vi "SimulationSubVI.vi"(0 "varIn":T1={"nodes"=[], "edges"=[], "nodeSelected"=-1, "bPressed"=FALSE, "NodeRef"=[]} {"edges"."len" format="%.2f"; "nodes"."h" format="%.2f"; "nodes"."w" format="%.2f"; "nodes"."dy" format="%.2f"; "nodes"."dx" format="%.2f"; "nodes"."y" format="%.2f"; "nodes"."x" format="%.2f"}) -> (14 "varOut":T1={"nodes"=[], "edges"=[], "nodeSelected"=-1, "bPressed"=FALSE, "NodeRef"=[]} {"edges"."len" format="%.2f"; "nodes"."h" format="%.2f"; "nodes"."w" format="%.2f"; "nodes"."dy" format="%.2f"; "nodes"."dx" format="%.2f"; "nodes"."y" format="%.2f"; "nodes"."x" format="%.2f"})   [LabVIEW 2010]
uses:
  localVar.ctl
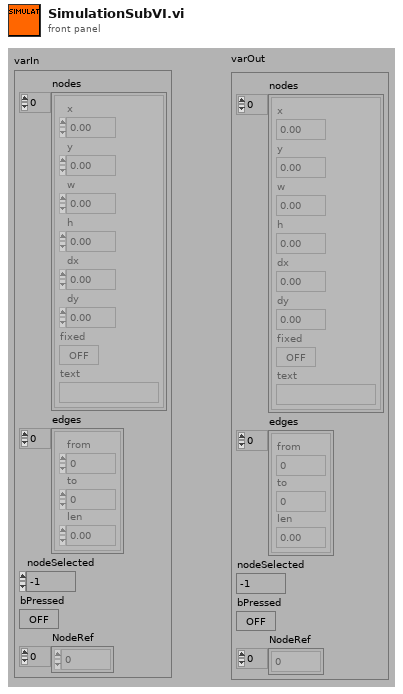
[diagram p1: front panel]
types:
  T1 = typedef "localVar.ctl" = cluster{"nodes":cluster{"x":dbl, "y":dbl, "w":dbl, "h":dbl, "dx":dbl, "dy":dbl, "fixed":bool, "text":string}[], "edges":cluster{"from":i32, "to":i32, "len":dbl}[], "nodeSelected":i32, "bPressed":bool, "NodeRef":u32[]}
  T2 = cluster{"x":dbl, "y":dbl, "w":dbl, "h":dbl, "dx":dbl, "dy":dbl, "fixed":bool, "text":string}[]
  T3 = cluster{"x":dbl, "y":dbl, "w":dbl, "h":dbl, "dx":dbl, "dy":dbl, "fixed":bool, "text":string}
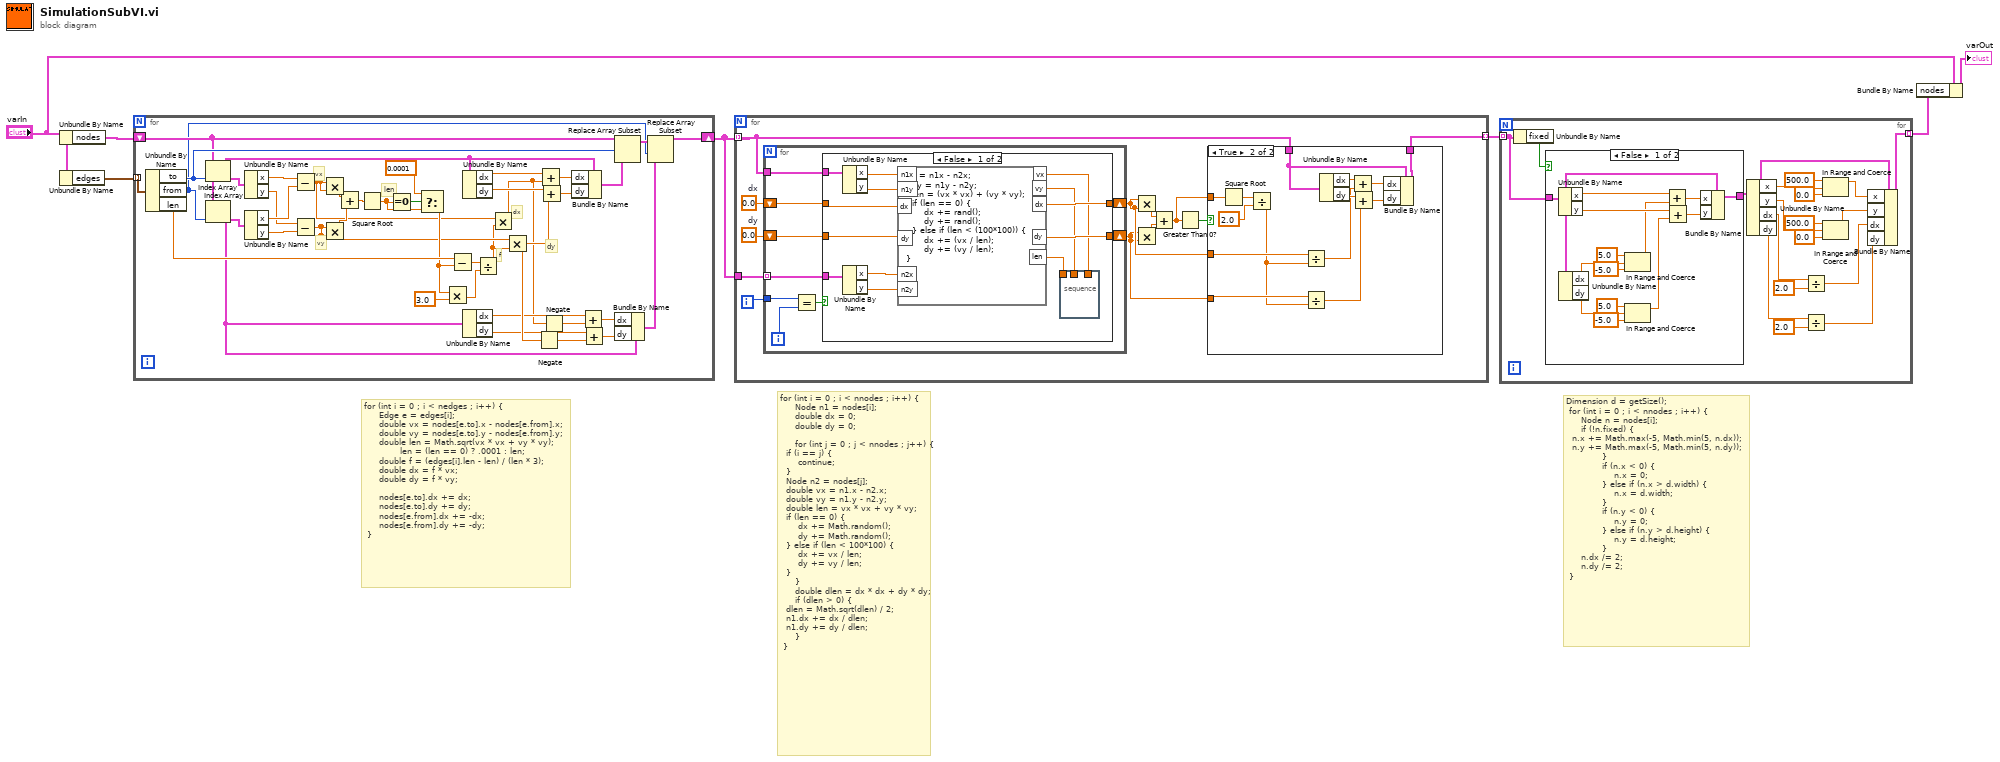
[diagram p0: block diagram]
diagram:
  # "Dimension d = getSize();\n\tfor (int i = 0 ; i < nnodes ; i++) {\n\t    Node n = nodes[i];\n\t    if (!n.fixed) {\n\t\tn.x += Math.max(-5, Math.min(5, n.dx));\n\t\tn.y += Math.max(-5, Math.min(5, n.dy));\n            }\n            if (n.x < 0) {\n                n.x = 0;\n            } else if (n.x > d.width) {\n                n.x = d.width;\n            }\n            if (n.y < 0) {\n                n.y = 0;\n            } else if (n.y > d.height) {\n                n.y = d.height;\n            }\n\t    n.dx /= 2;\n\t    n.dy /= 2;\n\t}"
  # "for (int i = 0 ; i < nnodes ; i++) {\n\t    Node n1 = nodes[i];\n\t    double dx = 0;\n\t    double dy = 0;\n\n\t    for (int j = 0 ; j < nnodes ; j++) {\n\t\tif (i == j) {\n\t\t    continue;\n\t\t}\n\t\tNode n2 = nodes[j];\n\t\tdouble vx = n1.x - n2.x;\n\t\tdouble vy = n1.y - n2.y;\n\t\tdouble len = vx * vx + vy * vy;\n\t\tif (len == 0) {\n\t\t    dx += Math.random();\n\t\t    dy += Math.random();\n\t\t} else if (len < 100*100) {\n\t\t    dx += vx / len;\n\t\t    dy += vy / len;\n\t\t}\n\t    }\n\t    double dlen = dx * dx + dy * dy;\n\t    if (dlen > 0) {\n\t\tdlen = Math.sqrt(dlen) / 2;\n\t\tn1.dx += dx / dlen;\n\t\tn1.dy += dy / dlen;\n\t    }\n\t}"
  # "for (int i = 0 ; i < nedges ; i++) {\n\t    Edge e = edges[i];\n\t    double vx = nodes[e.to].x - nodes[e.from].x;\n\t    double vy = nodes[e.to].y - nodes[e.from].y;\n\t    double len = Math.sqrt(vx * vx + vy * vy);\n            len = (len == 0) ? .0001 : len;\n\t    double f = (edges[i].len - len) / (len * 3);\n\t    double dx = f * vx;\n\t    double dy = f * vy;\n\n\t    nodes[e.to].dx += dx;\n\t    nodes[e.to].dy += dy;\n\t    nodes[e.from].dx += -dx;\n\t    nodes[e.from].dy += -dy;\n\t}"
  n1 = Unbundle By Name("varIn") -> ("nodes"=w6:T2)
  n2 = Unbundle By Name("varIn") -> ("edges"=w7:cluster{"from":i32, "to":i32, "len":dbl}[])
  n3 = for {
    tunnel: w7 -> [w47] mode=indexing
    shift-right: [w12] -> w1
    shift-left: w6 -> [w15]
    # "dy"
    # "dx"
    # "f"
    # "len"
    # "vy"
    # "vx"
    n4 = Unbundle By Name(w47) -> ("to"=w16:i32, "from"=w11:i32, "len"=w36:dbl)
    n5 = Index Array(array=w15, index=w16) -> (element=w31:T3)
    n6 = Index Array(array=w15, index=w11) -> (element=w17:T3)
    n7 = Unbundle By Name(w31) -> ("x"=w46:dbl, "y"=w43:dbl)
    n8 = Unbundle By Name(w17) -> ("x"=w45:dbl, "y"=w44:dbl)
    n9 = Subtract(x=w46, y=w45) -> (x-y=w26:dbl)
    n10 = Subtract(x=w43, y=w44) -> (x-y=w25:dbl)
    n11 = Multiply(x=w26, y=w26) -> (x*y=w41:dbl)
    n12 = Multiply(x=w25, y=w25) -> (x*y=w42:dbl)
    n13 = Add(x=w41, y=w42) -> (x+y=w40:dbl)
    n14 = Square Root(x=w40) -> (sqrt(x)=w37:dbl)
    n15 = Equal To 0?(x=w37) -> (x = 0?=w39:bool)
    n16 = Select(t=0.0001, s=w39, f=w37) -> (s? t:f=w34:dbl)
    n17 = Multiply(x=w34, y=3.0) -> (x*y=w32:dbl)
    n18 = Subtract(x=w36, y=w34) -> (x-y=w35:dbl)
    n19 = Unbundle By Name(w31) -> ("dx"=w30:dbl, "dy"=w29:dbl)
    n20 = Unbundle By Name(w17) -> ("dx"=w20:dbl, "dy"=w19:dbl)
    n21 = Divide(x=w35, y=w32) -> (x/y=w24:dbl)
    n22 = Multiply(x=w26, y=w24) -> (x*y=w18:dbl)
    n23 = Multiply(x=w25, y=w24) -> (x*y=w23:dbl)
    n24 = Negate(x=w23) -> (-x=w8:dbl)
    n25 = Add(x=w30, y=w18) -> (x+y=w28:dbl)
    n26 = Add(x=w29, y=w23) -> (x+y=w27:dbl)
    n27 = Negate(x=w18) -> (-x=w9:dbl)
    n28 = Bundle By Name(cluster=w31, "dx"=w28, "dy"=w27) -> (w14:T3)
    n29 = Add(x=w20, y=w9) -> (x+y=w21:dbl)
    n30 = Add(x=w19, y=w8) -> (x+y=w22:dbl)
    n31 = Replace Array Subset(array=w15, new element=w14, index=w16) -> (w13:T2)
    n32 = Bundle By Name(cluster=w17, "dx"=w21, "dy"=w22) -> (w10:T3)
    n33 = Replace Array Subset(array=w13, new element=w10, index=w11) -> (w12:T2)
  }
  n34 = for {
    tunnel: w1 -> [w48] mode=indexing
    tunnel: [w52] -> w3 mode=indexing
    tunnel: w1 -> [w49]
    i -> [w59]
    w58 = 0.0  # dx
    w57 = 0.0  # dy
    n35 = for {
      tunnel: w59 -> [w83]
      shift-right: [w80] -> w51
      shift-left: w58 -> [w79]
      shift-right: [w78] -> w50
      shift-left: w57 -> [w77]
      tunnel: w49 -> [w76] mode=indexing
      tunnel: w48 -> [w75]
      i -> [w82]
      n36 = Equal?(x=w83, y=w82) -> (x = y?=w81:bool)
      n37 = case shown="False" w81 {
        tunnel: [w87 w98] -> w80
        tunnel: w79 -> [w92 w98]
        tunnel: [w88 w97] -> w78
        tunnel: w77 -> [w89 w97]
        tunnel: w76 -> [w95 _]
        tunnel: w75 -> [w96 _]
        frame False {
          n38 = Unbundle By Name(w96) -> ("x"=w94:dbl, "y"=w93:dbl)
          n39 = Unbundle By Name(w95) -> ("x"=w90:dbl, "y"=w91:dbl)
          n40 = formula code="vx = n1x - n2x;\n\t\tvy = n1y - n2y;\n\t\tlen = (vx * vx) + (vy * vy);\n\t\tif (len == 0) {\n\t\t    dx += rand();\n\t\t    dy += rand();\n\t\t} else if (len < (100*100)) {\n\t\t    dx += (vx / len);\n\t\t    dy += (vy / len);\n}"("n1x"=w94, "n1y"=w93, "n2x"=w90, "n2y"=w91, "dx"=w92, "dy"=w89) -> ("vx"=w84:dbl, "vy"=w85:dbl, "dx"=w87:dbl, "dy"=w88:dbl, "len"=w86:dbl)
          n41 = stacked-sequence {
            tunnel: w86 -> [_]
            tunnel: w85 -> [_]
            tunnel: w84 -> [_]
            frame #0 {
            }
          }
        }
        frame True {
          # "SKIP"
        }
      }
    }
    n42 = Multiply(x=w51, y=w51) -> (x*y=w56:dbl)
    n43 = Multiply(x=w50, y=w50) -> (x*y=w55:dbl)
    n44 = Add(x=w56, y=w55) -> (x+y=w53:dbl)
    n45 = Greater Than 0?(x=w53) -> (x > 0?=w54:bool)
    n46 = case shown="True" w54 {
      tunnel: w53 -> [_ w74]
      tunnel: w48 -> [w60 w67]
      tunnel: [w60 w66] -> w52
      tunnel: w51 -> [_ w65]
      tunnel: w50 -> [_ w64]
      frame False {
      }
      frame True {
        n47 = Square Root(x=w74) -> (sqrt(x)=w73:dbl)
        n48 = Divide(x=w73, y=2.0) -> (x/y=w63:dbl)
        n49 = Divide(x=w65, y=w63) -> (x/y=w62:dbl)
        n50 = Divide(x=w64, y=w63) -> (x/y=w61:dbl)
        n51 = Unbundle By Name(w67) -> ("dx"=w70:dbl, "dy"=w71:dbl)
        n52 = Add(x=w70, y=w62) -> (x+y=w69:dbl)
        n53 = Add(x=w71, y=w61) -> (x+y=w68:dbl)
        n54 = Bundle By Name(cluster=w67, "dx"=w69, "dy"=w68) -> (w66:T3)
      }
    }
  }
  n55 = for {
    tunnel: w3 -> [w115] mode=indexing
    tunnel: [w99] -> w2 mode=indexing
    n56 = Unbundle By Name(w115) -> ("fixed"=w116:bool)
    n57 = case shown="False" w116 {
      tunnel: w115 -> [w122 w131]
      tunnel: [w117 w131] -> w106
      frame False {
        n58 = Unbundle By Name(w122) -> ("x"=w128:dbl, "y"=w127:dbl)
        n59 = Unbundle By Name(w122) -> ("dx"=w126:dbl, "dy"=w119:dbl)
        n60 = In Range and Coerce(upper limit=5.0, x=w126, lower limit=-5.0) -> (coerced(x)=w123:dbl)  [unwired: 1 out]
        n61 = In Range and Coerce(upper limit=5.0, x=w119, lower limit=-5.0) -> (coerced(x)=w118:dbl)  [unwired: 1 out]
        n62 = Add(x=w128, y=w123) -> (x+y=w129:dbl)
        n63 = Add(x=w127, y=w118) -> (x+y=w130:dbl)
        n64 = Bundle By Name(cluster=w122, "x"=w129, "y"=w130) -> (w117:T3)
      }
      frame True {
      }
    }
    n65 = Unbundle By Name(w106) -> ("x"=w114:dbl, "y"=w109:dbl, "dx"=w105:dbl, "dy"=w102:dbl)
    n66 = Divide(x=w105, y=2.0) -> (x/y=w100:dbl)
    n67 = Divide(x=w102, y=2.0) -> (x/y=w101:dbl)
    n68 = In Range and Coerce(upper limit=500.0, x=w114, lower limit=0.0) -> (coerced(x)=w108:dbl)  [unwired: 1 out]
    n69 = In Range and Coerce(upper limit=500.0, x=w109, lower limit=0.0) -> (coerced(x)=w107:dbl)  [unwired: 1 out]
    n70 = Bundle By Name(cluster=w106, "x"=w108, "y"=w107, "dx"=w100, "dy"=w101) -> (w99:T3)
  }
  n71 = Bundle By Name(cluster="varIn", "nodes"=w2) -> (→"varOut":T1)
